vi "Execute Laser Off.vi"(8 "error in":errorcluster, 11 "TSI 3025 in":refnum<class "TSI 3025.lvclass">) -> (0 "error out":errorcluster, 2 "CMD Good":bool, 3 "TSI 3025 out":refnum<class "TSI 3025.lvclass">)   [LabVIEW 2014, in "TSI 3025.lvclass"]
uses:
  TSI 3025.lvclass
  CPC.lvclass/CPC.ctl
  Accessors/Read Session Handle.vi
  Accessors/Write Session Handle.vi
  reusable/Session APIs/Serial/Public/Get Data/Get String.vi
  reusable/Session APIs/Serial/Serial Session.lvclass
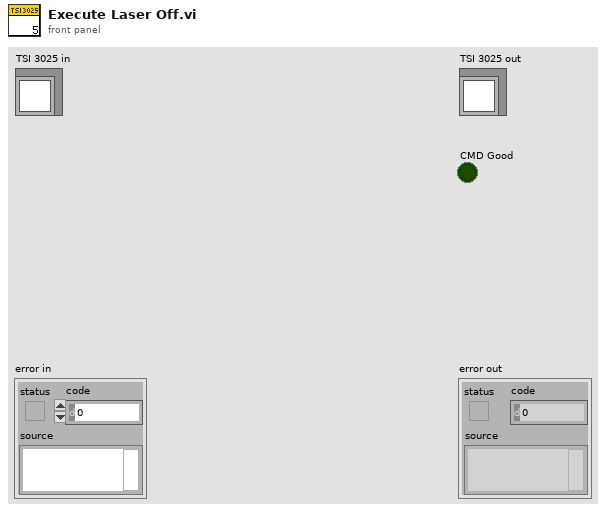
[diagram p1: front panel]
types:
  T1 = typedef "Serial Session.lvclass/Session Handle.ctl" = refnum<data-value>
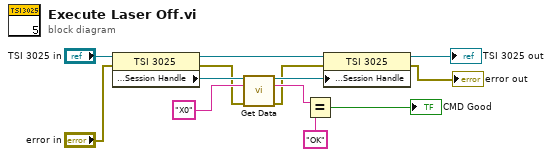
[diagram p0: block diagram]
diagram:
  n1 = property class="TSI 3025"(reference="TSI 3025 in", error in="error in") -> (reference out=w6:refnum<class "TSI 3025.lvclass">, error out=w1:errorcluster, "Accessors:Session Handle"=w10:T1)
  n2 = call-poly "Get Data.vi"("Session Handle in"=w10, "CMD"="X0" ("string"), "error in"=w1) -> ("Session Handle out"=w7:T1, "DataOut"=w9:string, "error out"=w4:errorcluster)  [unwired: 10 in]
  n3 = Equal?(x=w9, y="OK") -> (x = y?=→"CMD Good":bool)
  n4 = property class="TSI 3025"(reference=w6, error in=w4, "Accessors:Session Handle"=w7) -> (reference out=→"TSI 3025 out":refnum<class "TSI 3025.lvclass">, error out=→"error out":errorcluster)
